vi "Project Launcher.vi"() -> ()   [LabVIEW 2018]
doc: "This is the top-level VI of this application. When it runs, it behaves like the splash screen many applications use to keep the user occupied while the application loads into memory. This application is quite small, so there is little overhead, which would make the splash screen just flash for a moment. Because that flash is distracting, there is a three-second delay inserted into this VI so that it stays up for a little bit. \n\nThis VI uses a delay-loaded subVI call to load the rest of the application. This trick ensures that the splash screen can load instantly regardless of how large the rest of the VI hierarchy gets, and the loading of the rest of the VIs becomes one step in the load process."
uses:
  ADM/ADM/Load App.vi
  ADM/ADM/Main.lvclass
panel:
  out "Application Name":string
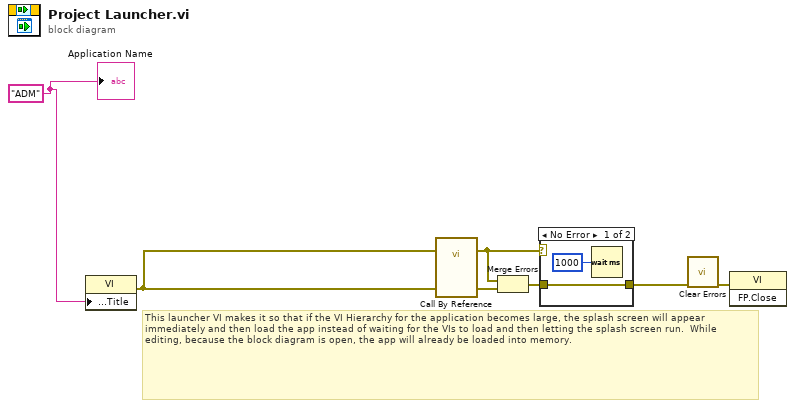
[diagram p0: block diagram]
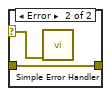
[diagram p2: hidden frame]
diagram:
  w1 = "ADM" ("Application Name")
  # "This launcher VI makes it so that if the VI Hierarchy for the application becomes large, the splash screen will appear immediately and then load the app instead of waiting for the VIs to load and then letting the splash screen run.  While editing, because the block diagram is open, the app will already be loaded into memory."
  n1 = property class="VI"("Front Panel.Title"=w1) -> (error out=w7:errorcluster)  [unwired: 2 in, 1 out]
  n2 = call-by-ref "?"(error in=w7, 8:"error in (no error)"=w7) -> (error out=w3:errorcluster, 0:"error out"=w6:errorcluster)  [unwired: 11 in, 1 out]
  n3 = Merge Errors(w3, w6) -> (w4:errorcluster)
  n4 = case shown="No Error" w3 {
    tunnel: [w9 w10] -> w2
    tunnel: w4 -> [w9 w10]
    selector: w3 -> [_ w11]
    frame No Error {
      n5 = Wait (ms)(milliseconds to wait=u32 1000) -> ()  [unwired: 1 out]
    }
    frame Error {
      n6 = call <vilib>:"Simple Error Handler.vi"("error in (no error)"=w11) -> ()  [unwired: 4 in, 5 out]
    }
  }
  n7 = call <vilib>:"Clear Errors.vi"("error in (no error)"=w2) -> ("error out"=w5:errorcluster)  [unwired: 5 in, 1 out]
  n8 = invoke class="VI" method="FP.Close"(error in=w5) -> ()  [unwired: 2 in, 3 out]
  "Application Name" <- w1
